vi "uartGetFrame.vi"   [LabVIEW 2020]
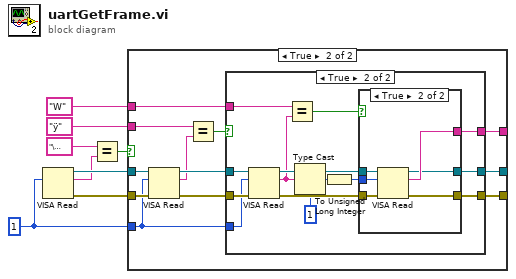
[diagram p0: block diagram]
diagram:
  w6 = u32 1 ("byte count")
  n1 = VISA Read(byte count=w6) -> (VISA resource name out=w8:refnum<visa-resource-name>, read buffer=w5:string, error out=w7:errorcluster)  [unwired: 2 in, 1 out]
  n2 = Equal?(x="\u0002" ("y"), y=w5) -> (x = y?=w3:bool)
  n3 = case shown="True" w3 {
    tunnel: w8 -> [w9 w22]
    tunnel: w7 -> [w10 w19]
    tunnel: w6 -> [_ w18]
    tunnel: "ÿ" ("y") -> [_ w16]
    tunnel: "W" ("y") -> [_ w14]
    tunnel: [_ w13] -> _
    tunnel: [w9 w12] -> _
    tunnel: [w10 w11] -> _
    frame False {
    }
    frame True {
      n4 = VISA Read(VISA resource name=w22, byte count=w18, error in (no error)=w19) -> (VISA resource name out=w21:refnum<visa-resource-name>, read buffer=w17:string, error out=w20:errorcluster)  [unwired: 1 out]
      n5 = Equal?(x=w16, y=w17) -> (x = y?=w15:bool)
      n6 = case shown="True" w15 {
        tunnel: w21 -> [w24 w38]
        tunnel: w20 -> [w23 w36]
        tunnel: w18 -> [_ w35]
        tunnel: w14 -> [_ w34]
        tunnel: [_ w27] -> w13
        tunnel: [w24 w26] -> w12
        tunnel: [w23 w25] -> w11
        frame False {
        }
        frame True {
          n7 = VISA Read(VISA resource name=w38, byte count=w35, error in (no error)=w36) -> (VISA resource name out=w37:refnum<visa-resource-name>, read buffer=w31:string, error out=w33:errorcluster)  [unwired: 1 out]
          n8 = Equal?(x=w34, y=w31) -> (x = y?=w32:bool)
          n9 = Type Cast(type=u8 1 ("byte count"), x=w31) -> (*(type *) &x=w29:u8)
          n10 = To Unsigned Long Integer(number=w29) -> (unsigned 32bit integer=w28:u32)
          n11 = case shown="True" w32 {
            tunnel: w37 -> [w40 w46]
            tunnel: w33 -> [w39 w45]
            tunnel: w28 -> [_ w44]
            tunnel: [_ w43] -> w27
            tunnel: [w40 w42] -> w26
            tunnel: [w39 w41] -> w25
            frame False {
            }
            frame True {
              n12 = VISA Read(VISA resource name=w46, byte count=w44, error in (no error)=w45) -> (VISA resource name out=w42:refnum<visa-resource-name>, read buffer=w43:string, error out=w41:errorcluster)  [unwired: 1 out]
            }
          }
        }
      }
    }
  }
